vi "Find Block Diagram Resource.vi"(8 "error in (no error)":errorcluster, 11 "Resources":T1[](array[typedef])) -> (0 "error out":errorcluster, 1 "Index":i32, 2 "Resource":T1, 3 "Resources out":T1[](array[typedef]), 5 "Found?":bool)   [LabVIEW 2026, in "VILab.lvlib"]
uses:
  VILab.lvlib
  CTLs/Resource.ctl
  Find First Matching Resource (String).vi
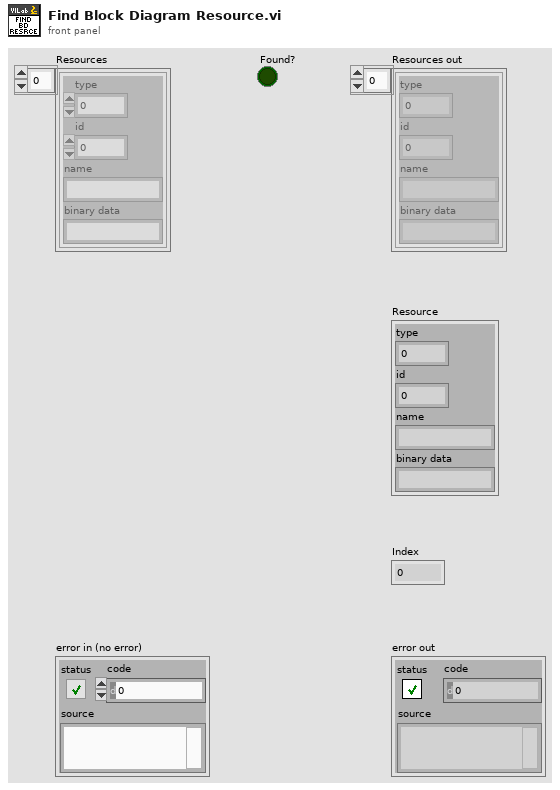
[diagram p1: front panel]
types:
  T1 = typedef "VILab.lvlib/Resource.ctl" = cluster{"type":u32, "id":i32, "name":string, "binary data":string}
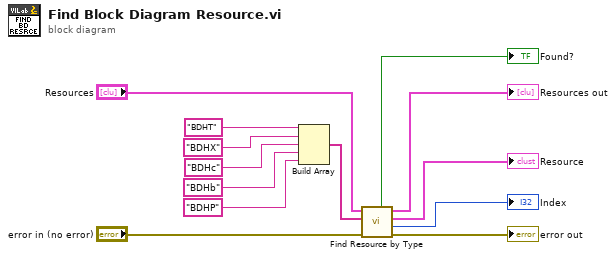
[diagram p0: block diagram]
diagram:
  n1 = Build Array("BDHT", "BDHX", "BDHc", "BDHb", "BDHP") -> (w2:string[])
  n2 = call-poly "Find Resource by Type.vi"("error in (no error)"="error in (no error)", "Resource Types"=w2, "Resources"="Resources") -> ("error out"=→"error out":errorcluster, "Index"=→"Index":i32, "Resource"=→"Resource":T1, "Resources out"=→"Resources out":T1[], "Found?"=→"Found?":bool)  [unwired: 4 in]
